vi "Find Largest Common Substring.vi"(9 "String 2":string, 11 "String 1":string) -> (0 "Start Index 2":i32, 1 "Start Index 1":i32, 2 "Largest Common String":string)   [LabVIEW 2021, in "Strings.lvlib"]
uses:
  Strings.lvlib
  Time/Time.lvlib
panel:
  out "CPU (ms)":dbl
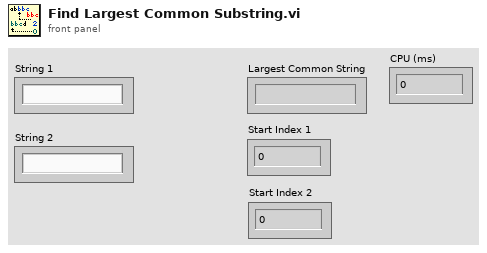
[diagram p1: front panel]
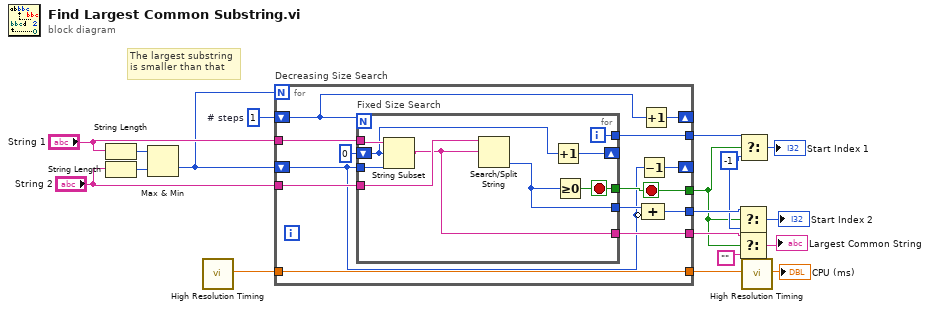
[diagram p0: block diagram]
diagram:
  w8 = -1 ("f")
  w13 = 1  # # steps
  # "The largest substring\nis smaller than that"
  n1 = String Length(string="String 1") -> (length=w18:i32)
  n2 = String Length(string="String 2") -> (length=w17:i32)
  n3 = Max & Min(x=w18, y=w17) -> (min(x,y)=w14:i32)  [unwired: 1 out]
  n4 = call "High Resolution Timing.vi"() -> ("elapsed (relative) seconds"=w3:dbl)  [unwired: 17 in, 2 out]
  n5 = for "Decreasing Size Search" {
    N: w14 -> [_]
    tunnel: "String 1" -> [w30]
    shift-right: [w26] -> _
    shift-left: w14 -> [w22]
    tunnel: "String 2" -> [w29]
    tunnel: [w23] -> w10
    tunnel: [w27] -> w7
    tunnel: [w25] -> w6
    tunnel: [w24] -> w12
    shift-right: [w20] -> _
    shift-left: w13 -> [w21]
    tunnel: w3 -> [w19]
    tunnel: [w19] -> w2
    stop <- w25 stop-if-true
    n6 = for "Fixed Size Search" {
      N: w21 -> [_]
      shift-right: [w37] -> _
      shift-left: 0 -> [w38]
      tunnel: w30 -> [w40]
      tunnel: w22 -> [w39]
      tunnel: w29 -> [w34]
      tunnel: [w32] -> w28
      tunnel: [w33] -> w27
      tunnel: [w36] -> w25
      tunnel: [w35] -> w24
      i -> [w35]
      stop <- w36 stop-if-true
      n7 = String Subset(string=w40, offset (0)=w38, length (rest)=w39) -> (substring=w33:string)
      n8 = Search/Split String(string=w34, search string/char (-)=w33) -> (offset of match=w32:i32)  [unwired: 1 in, 2 out]
      n9 = Increment(x=w38) -> (x+1=w37:i32)
      n10 = Greater Or Equal To 0?(x=w32) -> (x >= 0?=w36:bool)
    }
    n11 = Decrement(x=w22) -> (x-1=w26:i32)
    n12 = Increment(x=w21) -> (x+1=w20:i32)
    n13 = Compound Arithmetic op=ADD(w28, invert w22) -> (w23:i32)
  }
  n14 = Select(t=w10, s=w6, f=w8) -> (s? t:f=→"Start Index 2":i32)
  n15 = Select(t=w7, s=w6, f="") -> (s? t:f=→"Largest Common String":string)
  n16 = Select(t=w12, s=w6, f=w8) -> (s? t:f=→"Start Index 1":i32)
  n17 = call "High Resolution Timing.vi"("relative seconds (NaN)"=w2) -> ("elapsed (relative) seconds"=→"CPU (ms)":dbl)  [unwired: 16 in, 2 out]
